vi "PH_gentec_Powermeter.panel.vi"(0 "object ref":refnum<vi>, 5 "error in (no error)":errorcluster) -> (19 "error out":errorcluster)   [LabVIEW 2014, in "PH_gentec_Powermeter.lvlib"]
doc: "By this VI apowermeter can be operated. \n\nThe panel is divided into the Tab Control which contains three pages and the most important elements.\nThe 1st page of the Tab Control contains the general information Range, Trigger Level, Scaling Factor (the user can set these values), Uncorrected Value and Serial Number (these are indicators). \nThe 2nd page contains everything relevant for the Statistics Mode of the powermeter. Here you can Start/Stop the statistic data collection, set the Number of Pulses, Percentage of Pulses and the Number of Samples. The Cluster 'Statistic Data' views the evaluated statistic data.\nThe 3rd page contains the rarely needed status-information of the powermeter. The string views data like Active Sensitivity, Offset, Resolution and so on.\n\nBelow the Tab Control you can see: \n - Current Value views the value that is currently being displayed on the device's screen. The correct unit is appended.\n - Powermeter views the Device State: blue means no info\n darkgreen means off\n lightgreen means operating\n yellow means error detected\n - EXIT closes the front panel (GUI), while\n - Delete Instance disconnects and removes the instance from the PCS.\n\n\nLicense Agreement for this software:\n\nCopyright (C)\nGesellschaft für Schwerionenforschung, GSI\nPlanckstr. 1\n64291 Darmstadt\nGermany\n\nContact: D.Beck@gsi.de \n\nThis program is free software; you can redistribute it and/or modify it under the terms of the GNU General Public License as published by the Free Software Foundation; either version 2 of the license, or (at your option) any later version.\n\nThis program is distributed in the hope that it will be useful, but WITHOUT ANYW ARRANTY; without even the implied warranty of MERCHANTABILITY or FITNESS FOR A PARTICULAR PURPOSE. See the GNU General License for more details (http://www.gnu.org).\n\nGesellschaft für Schwerionenforschung, GSI\nPlanckstr. 1, 64291 Darmstadt, Germany\nFor all questions and ideas contact: M.Richter@gsi.de, H.Brand@gsi.de or D.Beck@gsi.de.\nLast update: 18-DEC-2002"
uses:
  PH_gentec_Powermeter.lvlib
  PH_StatusHandler/PH_StatusHandler.GUI element.ctl
  PH_Powermeter_BaseClass/PH_Powermeter_BaseClass.Energy.ctl
  PH_Powermeter_BaseClass/PH_Powermeter_BaseClass.Head Attributes.ctl
  PH_Powermeter_BaseClass/PH_Powermeter_BaseClass.Connection.ctl
  PH_Powermeter_BaseClass/PH_Powermeter_BaseClass.State.ctl
  non_GPL/instr.lib/gentec-SOLO-PE/Driver/Type Defs/gentec-SOLO-PE.Configuration Values.ctl
  non_GPL/instr.lib/gentec-SOLO-PE/Driver/Type Defs/gentec-SOLO-PE.Scale.ctl
  non_GPL/instr.lib/gentec-SOLO-PE/Driver/Type Defs/gentec-SOLO-PE.Statistics Data.ctl
  non_GPL/instr.lib/gentec-SOLO-PE/Driver/Type Defs/gentec-SOLO-PE.Data Sampling Settings.ctl
  PH_gentec_Powermeter.Sets.ctl
  PH_Powermeter_BaseClass/PH_gentec_BaseClass.Head Settings.ctl
  PH_Powermeter_BaseClass/PH_Powermeter_BaseClass.GUI Refs.ctl
  CSCore/CSObj/CSObj.lvlib
  CSCore/CSSystem/CSSystemLib/CSSystemLib.lvlib
  PH_Common/PH_Common.lvlib
  PH_Class/PH_Class.lvlib
  PH_Powermeter_BaseClass/PH_Powermeter_BaseClass.lvlib
  PH_StatusHandler/PH_StatusHandler.lvlib
  non_GPL/instr.lib/gentec-SOLO-PE/gentec-SOLO-PE - Driver.lvlib
panel:
  out "Status":T1
  out "PSDB Status":u32(colorbox)=6618880 caption="PSDB"
  in  "Tab Control":T2(tab)
  in  "Scaling Factor":dbl=1.0
  in  "Range":u32(ring) items=["Scale 1", "Scale 2", "Scale 3"]
  in  "Wavelength":u32=1 caption="nm"
  in  "Trigger Level":dbl caption="%"
  in  "Set Zero":bool
  out "Energy evolution":dbl(graph)
  out "Energy":T3={"current Value"=0.0, "unscaled"=0.0, "Scaling Factor"=1.0} {"unscaled" format="%#_6p"; "current Value" format="%#.1p"}
  in  "Start/Stop Statistics":bool caption="Start/Stop"
  in  "Data Sampling Settings":T4 {"Time Stamp" items=["Off", "On"]; "Total Duration Unit" items=["Period", "Seconds", "Minutes", "Hours", "Days", "Weeks", "Continuous", "# of Points"]; "Total Duration" max=300 step=1; "Sample Period Unit" items=["Seconds", "Minutes", "Hours", "Days", "Weeks", "Pulses"]; "Sample Rate Unit" items=["per Second", "per Minute", "per Hour", "per Day", "% pulses"]; "Sample Rate" max=300 step=1}
  out "Statistic Data":T5 {"Uncorrected Value" format="%.6f"; "Rep Rate" format="%.2f"; "Average Power" format="%.6f"; "PTP Stability" format="%.6f"; "RMS Stability" format="%.6f"; "Standard Deviation" format="%.6f"; "Average" format="%.6f"; "Minimum" format="%.6f"; "Maximum" format="%.6f"; "Current Value" format="%.6f"}
  out "Configuration Values":T6 {"Reference Value" format="%.6f"; "Lower Bond" format="%.6f"; "Upper Bound" format="%.6f"; "Resolution" format="%.7f"; "Max energy (Joulemeter)" format="%.6f"; "Max Power (Joulemeter)" format="%.6f"; "Offset 2" format="%.6f"; "Multiplier 2" format="%.6f"; "Offset 1" format="%.6f"; "Multiplier 1" format="%.6f"; "Zero Offset" format="%.6f"; "Trig Level" format="%.6f"; "Current Scale" items=["Auto", "1 pJ", "3 pJ", "10 pJ", "30 pJ", "100 pJ", "300 pJ", "1 nJ", "3 nJ", "10 nJ", "30 nJ", "100 nJ", "300 nJ", "1 uJ", "3 uJ", "10 uJ", "30 uJ", "100 uJ", "300 uJ", "1 mJ", "3 mJ", "10 mJ", "30 mJ", "100 mJ", "300 mJ", "1 J", "3 J", "10 J", "30 J", "100 J", "300 J", "1 kJ", "3 kJ", "10 kJ", "30 kJ", "100 kJ", "300 kJ", "1 MJ", "3 MJ", "10 MJ", "30 MJ", "100 MJ", "300 MJ"]; "Scale Max Energy" items=["Auto", "1 pJ", "3 pJ", "10 pJ", "30 pJ", "100 pJ", "300 pJ", "1 nJ", "3 nJ", "10 nJ", "30 nJ", "100 nJ", "300 nJ", "1 uJ", "3 uJ", "10 uJ", "30 uJ", "100 uJ", "300 uJ", "1 mJ", "3 mJ", "10 mJ", "30 mJ", "100 mJ", "300 mJ", "1 J", "3 J", "10 J", "30 J", "100 J", "300 J", "1 kJ", "3 kJ", "10 kJ", "30 kJ", "100 kJ", "300 kJ", "1 MJ", "3 MJ", "10 MJ", "30 MJ", "100 MJ", "300 MJ"]; "Scale Min Energy" items=["Auto", "1 pJ", "3 pJ", "10 pJ", "30 pJ", "100 pJ", "300 pJ", "1 nJ", "3 nJ", "10 nJ", "30 nJ", "100 nJ", "300 nJ", "1 uJ", "3 uJ", "10 uJ", "30 uJ", "100 uJ", "300 uJ", "1 mJ", "3 mJ", "10 mJ", "30 mJ", "100 mJ", "300 mJ", "1 J", "3 J", "10 J", "30 J", "100 J", "300 J", "1 kJ", "3 kJ", "10 kJ", "30 kJ", "100 kJ", "300 kJ", "1 MJ", "3 MJ", "10 MJ", "30 MJ", "100 MJ", "300 MJ"]; "Active Sensitivity" format="%.6f"; "Calibration Sensitivity" format="%.6f"}
  out "Current Settings":T8={"Trigger Level"=0.0, "Wavelength"=1, "Range"=0}
  out "Wanted Settings":T8={"Trigger Level"=0.0, "Wavelength"=1, "Range"=0}
  out "Wanted Sets":T9 {"Data Sampling Settings"."Time Stamp" items=["Off", "On"]; "Data Sampling Settings"."Total Duration Unit" items=["Period", "Seconds", "Minutes", "Hours", "Days", "Weeks", "Continuous", "# of Points"]; "Data Sampling Settings"."Total Duration" max=300 step=1; "Data Sampling Settings"."Sample Period Unit" items=["Seconds", "Minutes", "Hours", "Days", "Weeks", "Pulses"]; "Data Sampling Settings"."Sample Rate Unit" items=["per Second", "per Minute", "per Hour", "per Day", "% pulses"]; "Data Sampling Settings"."Sample Rate" max=300 step=1}
  out "Current Sets":T9 {"Data Sampling Settings"."Time Stamp" items=["Off", "On"]; "Data Sampling Settings"."Total Duration Unit" items=["Period", "Seconds", "Minutes", "Hours", "Days", "Weeks", "Continuous", "# of Points"]; "Data Sampling Settings"."Total Duration" max=300 step=1; "Data Sampling Settings"."Sample Period Unit" items=["Seconds", "Minutes", "Hours", "Days", "Weeks", "Pulses"]; "Data Sampling Settings"."Sample Rate Unit" items=["per Second", "per Minute", "per Hour", "per Day", "% pulses"]; "Data Sampling Settings"."Sample Rate" max=300 step=1}
  out "VISA resource":refnum<visa-resource-name>
  out "Connection":T10
  out "Head Attributes":T12={"Instrument Type"="---", "Head Version"="---", "Head Name"="---", "Serial Number"="---", "Firmware"="---", "Sensor Type"="---", "MinimumRange"=0, "Maximum Range"=0, "Min Wavelength"=-1, "Max Wavelength"=-1}
  in  "Delete":bool
  in  "Exit":bool
  # "PCS"
  # "3.40"
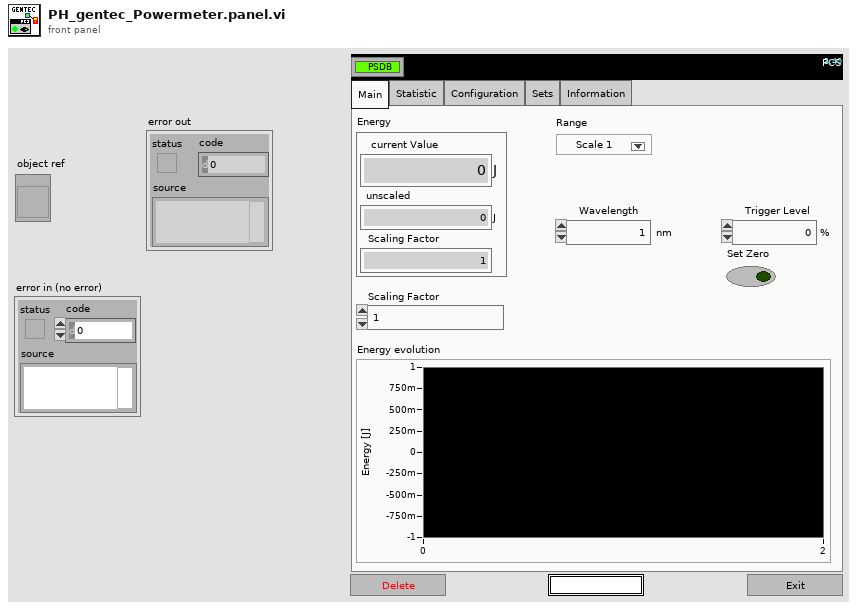
[diagram p1: front panel]
types:
  T1 = typedef "PH_StatusHandler.lvlib/PH_StatusHandler.GUI element.ctl" = u16
  T2 = enum32{"Main", "Statistic", "Configuration", "Sets", "Information"}
  T3 = typedef "PH_Powermeter_BaseClass.lvlib/PH_Powermeter_BaseClass.Energy.ctl" = cluster{"current Value":dbl, "unscaled":dbl, "Scaling Factor":dbl}
  T4 = typedef "gentec-SOLO-PE - Driver.lvlib/gentec-SOLO-PE.Data Sampling Settings.ctl" = cluster{"Sample Rate":u32, "Sample Rate Unit":u32, "Sample Period":u32, "Sample Period Unit":u32, "Total Duration":u32, "Total Duration Unit":u32, "Time Stamp":u32}
  T5 = typedef "gentec-SOLO-PE - Driver.lvlib/gentec-SOLO-PE.Statistics Data.ctl" = cluster{"Current Value":dbl, "Maximum":dbl, "Minimum":dbl, "Average":dbl, "Standard Deviation":dbl, "RMS Stability":dbl, "PTP Stability":dbl, "Current Time In Period":u32, "Total Time in Period":u32, "Pulse Number":u32, "Total Pulses":u32, "Average Power":dbl, "Rep Rate":dbl, "Uncorrected Value":dbl}
  T6 = typedef "gentec-SOLO-PE - Driver.lvlib/gentec-SOLO-PE.Configuration Values.ctl" = cluster{"Head Type":string, "Head Version":u32, "Serial Number":string, "Calibration Sensitivity":dbl, "Default Wavelength":u32, "Active Sensitivity":dbl, "Active Wavelength":u32, "Scale Min Power":u32, "Scale Max Power":u32, "Scale Min Energy":T7, "Scale Max Energy":T7, "Current Scale":T7, "Calo Mode":bool, "Anticipation":bool, "External Trig":bool, "Trig Level":dbl, "Zero Offset":dbl, "Multiplier 1":dbl, "Offset 1":dbl, "Multiplier 2":dbl, "Offset 2":dbl, "Max Power (Joulemeter)":dbl, "Max energy (Joulemeter)":dbl, "Currently Logging":bool, "Analog Out Active":bool, "Resolution":dbl, "Currently Calculating Stats":bool, "High-Resolution Display":bool, "Scale Min Wavelenght":u32, "Scale Max Wavelenght":u32, "Upper Bound":dbl, "Lower Bond":dbl, "Reference Value":dbl, "Thresholds Active":bool, "Fail":bool}
  T7 = typedef "gentec-SOLO-PE - Driver.lvlib/gentec-SOLO-PE.Scale.ctl" = u32
  T8 = typedef "PH_Powermeter_BaseClass.lvlib/PH_gentec_BaseClass.Head Settings.ctl" = cluster{"Trigger Level":dbl, "Wavelength":u32, "Range":u32}
  T9 = typedef "PH_gentec_Powermeter.lvlib/PH_gentec_Powermeter.Sets.ctl" = cluster{"Data Sampling Settings":T4, "Set Zero":bool}
  T10 = typedef "PH_Powermeter_BaseClass.lvlib/PH_Powermeter_BaseClass.Connection.ctl" = cluster{"failed checks":i8, "Timeout":bool, "Data read":string, "Failure":bool, "Error":bool, "State":T11}
  T11 = typedef "PH_Powermeter_BaseClass.lvlib/PH_Powermeter_BaseClass.State.ctl" = enum32{"off", "operating", "opened", "checked", "connected", "Sets to change", "running"}
  T12 = typedef "PH_Powermeter_BaseClass.lvlib/PH_Powermeter_BaseClass.Head Attributes.ctl" = cluster{"Instrument Type":string, "Head Version":string, "Head Name":string, "Serial Number":string, "Firmware":string, "Sensor Type":string, "MinimumRange":u32, "Maximum Range":u32, "Min Wavelength":i32, "Max Wavelength":i32}
  T13 = typedef "PH_Powermeter_BaseClass.lvlib/PH_Powermeter_BaseClass.GUI Refs.ctl" = cluster{"Head Attributes":refnum<vi>, "Energy":refnum<vi>, "Connection":refnum<vi>, "VISA Resource":refnum<vi>, "Energy evolution":refnum<vi>, "Scaling Factor":refnum<vi>, "Range":refnum<vi>, "Wavelength":refnum<vi>, "Trigger Level":refnum<vi>, "Wanted Settings":refnum<vi>, "Current Settings":refnum<vi>}
  T14 = typedef "PH_gentec_Powermeter.lvlib/PH_gentec_Powermeter.i attribute.ctl" = cluster{"GUI References":cluster{"delete":refnum<vi>, "start stop Statistics":refnum<vi>, "Statistic Data":refnum<vi>, "Configuration Values":refnum<vi>, "Set Zero":refnum<vi>, "Data Sampling Settings":refnum<vi>, "Wanted Sets":refnum<vi>, "Current Sets":refnum<vi>}, "Start Stop Statistics":bool, "Wanted Sets":T9, "Current Sets":T9}
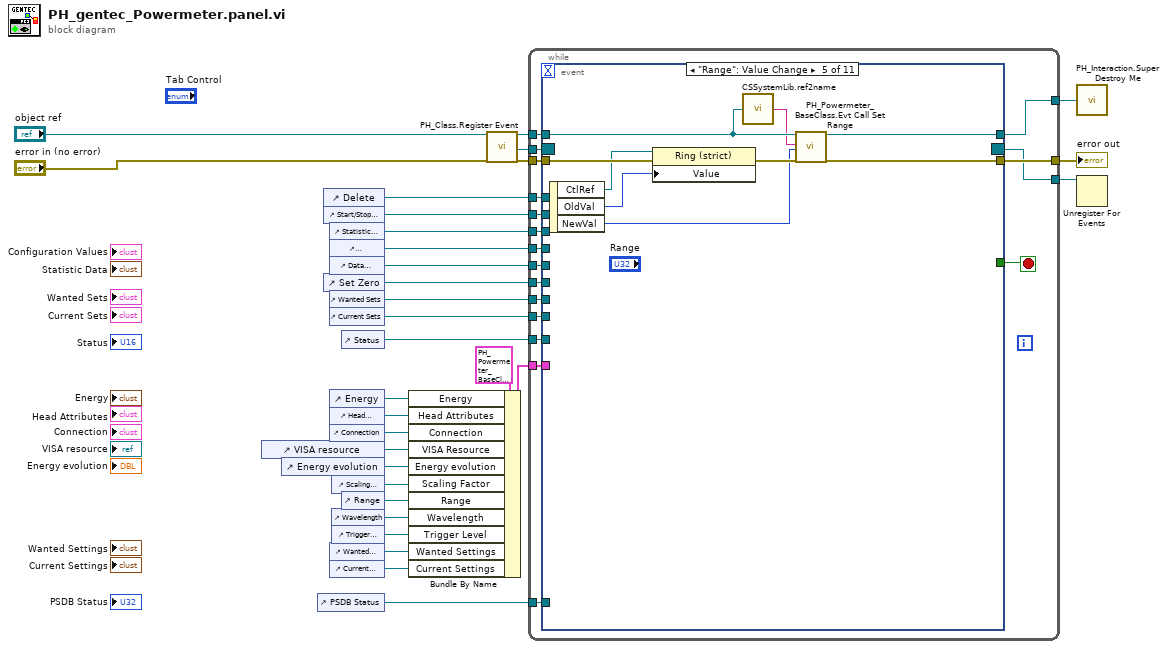
[diagram p0: block diagram]
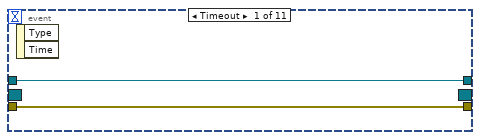
[diagram p2: hidden frame]
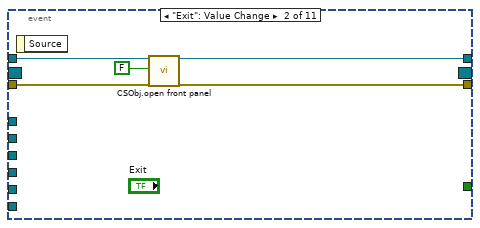
[diagram p3: hidden frame]
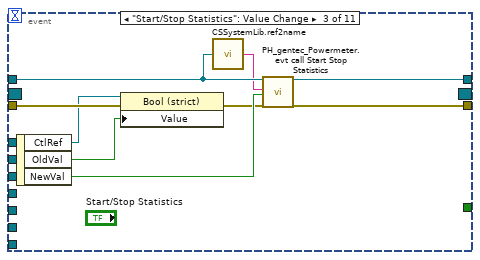
[diagram p4: hidden frame]
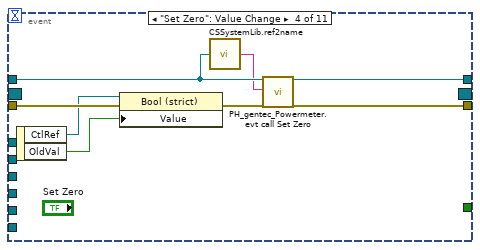
[diagram p5: hidden frame]
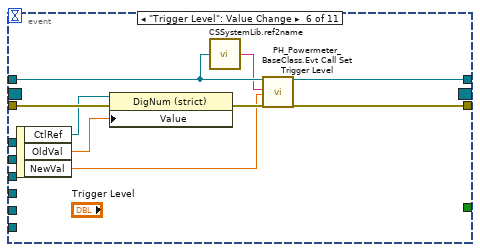
[diagram p6: hidden frame]
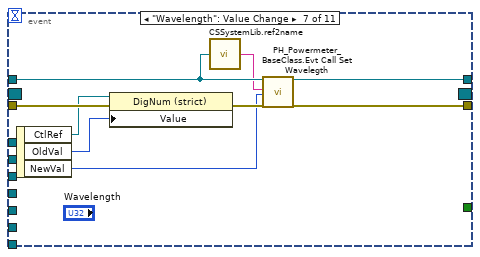
[diagram p7: hidden frame]
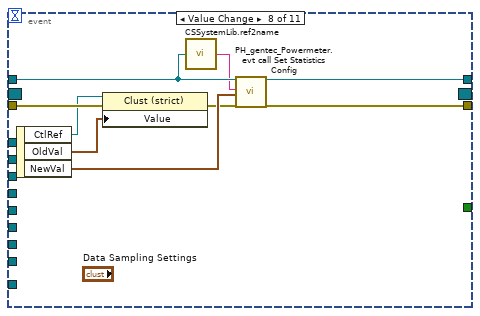
[diagram p8: hidden frame]
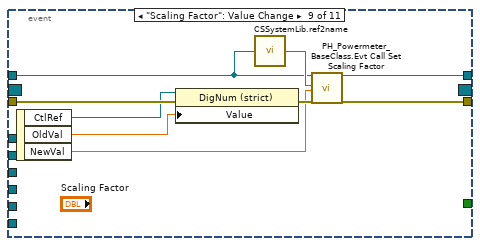
[diagram p9: hidden frame]
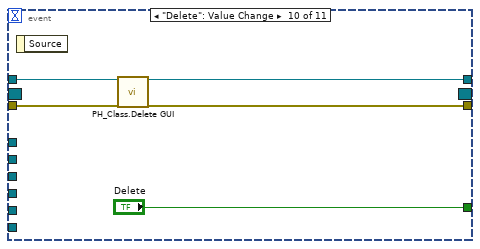
[diagram p10: hidden frame]
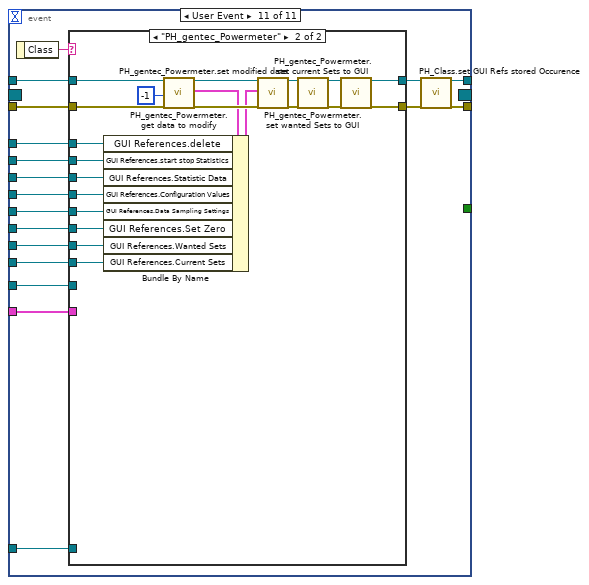
[diagram p11: hidden frame]
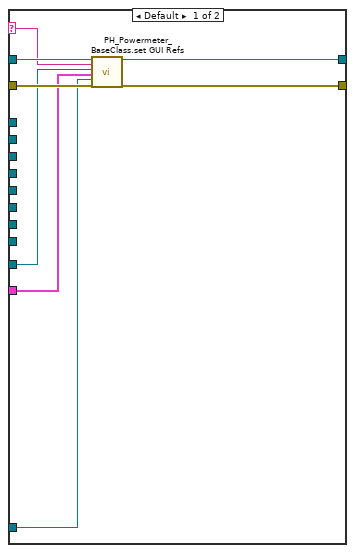
[diagram p12: hidden frame]
diagram:
  n1 = control-ref of="VISA resource"() -> (w14:refnum<vi>)
  n2 = control-ref of="Energy evolution"() -> (w9:refnum<vi>)
  n3 = control-ref of="PSDB Status"() -> (w21:refnum<vi>)
  n4 = control-ref of="Delete"() -> (w23:refnum<vi>)
  n5 = control-ref of="Start/Stop Statistics"() -> (w22:refnum<vi>)
  n6 = control-ref of="Set Zero"() -> (w13:refnum<vi>)
  n7 = control-ref of="Statistic Data"() -> (w12:refnum<vi>)
  n8 = control-ref of="Configuration Values"() -> (w11:refnum<vi>)
  n9 = control-ref of="Data Sampling Settings"() -> (w10:refnum<vi>)
  n10 = control-ref of="Wanted Sets"() -> (w2:refnum<vi>)
  n11 = control-ref of="Current Sets"() -> (w1:refnum<vi>)
  n12 = control-ref of="Energy"() -> (w17:refnum<vi>)
  n13 = control-ref of="Head Attributes"() -> (w16:refnum<vi>)
  n14 = control-ref of="Connection"() -> (w15:refnum<vi>)
  n15 = control-ref of="Wanted Settings"() -> (w7:refnum<vi>)
  n16 = control-ref of="Current Settings"() -> (w6:refnum<vi>)
  n17 = control-ref of="Scaling Factor"() -> (w8:refnum<vi>)
  n18 = control-ref of="Wavelength"() -> (w4:refnum<vi>)
  n19 = control-ref of="Trigger Level"() -> (w5:refnum<vi>)
  n20 = control-ref of="Status"() -> (w20:refnum<vi>)
  n21 = control-ref of="Range"() -> (w3:refnum<vi>)
  n22 = Bundle By Name(cluster=T13 {"Head Attributes"=refnum, "Energy"=refnum, "Connection"=refnum, "VISA Resource"=refnum, "Energy evolution"=refnum, "Scaling Factor"=refnum, "Range"=refnum, "Wavelength"=refnum, "Trigger Level"=refnum, "Wanted Settings"=refnum, "Current Settings"=refnum} ("Powermeter Base Class GUI References"), "Energy"=w17, "Head Attributes"=w16, "Connection"=w15, "VISA Resource"=w14, "Energy evolution"=w9, "Scaling Factor"=w8, "Range"=w3, "Wavelength"=w4, "Trigger Level"=w5, "Wanted Settings"=w7, "Current Settings"=w6) -> (w18:T13)
  n23 = call "PH_Class.Register Event.vi"("i ref in"="object ref", "error in (no error)"="error in (no error)") -> ("i ref out"=w29:refnum<vi>, "Event Registration Refnum"=w27:refnum<event-registration>, "error out"=w28:errorcluster)  [unwired: 15 in]
  n24 = while {
    tunnel: w29 -> [w46]
    tunnel: [w45] -> w30
    tunnel: w28 -> [w48]
    tunnel: [w47] -> w31
    tunnel: w27 -> [w44]
    tunnel: [w43] -> w26
    tunnel: w23 -> [w42]
    tunnel: w22 -> [w41]
    tunnel: w12 -> [w40]
    tunnel: w11 -> [w39]
    tunnel: w10 -> [w38]
    tunnel: w21 -> [w37]
    tunnel: w20 -> [w36]
    tunnel: w18 -> [w35]
    tunnel: w13 -> [w34]
    tunnel: w2 -> [w33]
    tunnel: w1 -> [w32]
    stop <- w49 stop-if-true
    n25 = event shown="[4] \"Range\": Value Change" {
      selector: w44 -> [_ _ _ _ _ _ _ _ _ _ _]
      dyn-events: [_ _ _ _ _ _ _ _ _ _ _] -> w43
      timeout: _ -> [_ _ _ _ _ _ _ _ _ _ _]
      tunnel: [_ _ _ _ _ _ _ _ _ "Delete" _] -> w49
      tunnel: w46 -> [w50 w56 w61 w71 w80 w89 w98 w106 w116 w121 w141]
      tunnel: w48 -> [w51 w54 w64 w69 w78 w87 w96 w109 w115 w122 w140]
      tunnel: [w51 w53 w63 w73 w82 w91 w100 w108 w114 w119 w136] -> w47
      tunnel: [w50 w52 w62 w72 w81 w90 w99 w107 w113 w120 w137] -> w45
      tunnel: w42 -> [_ _ _ _ _ _ _ _ _ _ w135]
      tunnel: w41 -> [_ _ _ _ _ _ _ _ _ _ w134]
      tunnel: w40 -> [_ _ _ _ _ _ _ _ _ _ w133]
      tunnel: w39 -> [_ _ _ _ _ _ _ _ _ _ w132]
      tunnel: w38 -> [_ _ _ _ _ _ _ _ _ _ w131]
      tunnel: w37 -> [_ _ _ _ _ _ _ _ _ _ w129]
      tunnel: w36 -> [_ _ _ _ _ _ _ _ _ _ w128]
      tunnel: w35 -> [_ _ _ _ _ _ _ _ _ _ w127]
      tunnel: w34 -> [_ _ _ _ _ _ _ _ _ _ w126]
      tunnel: w33 -> [_ _ _ _ _ _ _ _ _ _ w125]
      tunnel: w32 -> [_ _ _ _ _ _ _ _ _ _ w124]
      event Timeout {
        n26 = event-data() -> ()  [unwired: 1 in, 2 out]
      }
      event "Exit": Value Change {
        n27 = event-data() -> ()  [unwired: 1 in, 1 out]
        n28 = call "CSObj.open front panel.vi"("i ref in"=w56, "frontPanelOpen"=FALSE ("front panel open"), "error in (no error)"=w54) -> ("i ref out"=w52:refnum<vi>, "error out"=w53:errorcluster)  [unwired: 15 in]
      }
      event "Start/Stop Statistics": Value Change {
        n29 = event-data() -> ("CtlRef"=w58:refnum<vi>, "OldVal"=w57:bool, "NewVal"=w65:bool)  [unwired: 1 in]
        n30 = property class="Bool (strict)"(reference=w58, error in=w64, "Value"=w57) -> (error out=w59:errorcluster)  [unwired: 1 out]
        n31 = call "CSSystemLib.ref2name.vi"("obj refnum"=w61) -> ("name"=w60:string)
        n32 = call "PH_gentec_Powermeter.evt call Start Stop Statistics.vi"("i ref in"=w61, "Instance"=w60, "Start/Stop Statistics"=w65, "error in (no error)"=w59) -> ("i ref out"=w62:refnum<vi>, "error out"=w63:errorcluster)  [unwired: 14 in]
      }
      event "Set Zero": Value Change {
        n33 = event-data() -> ("CtlRef"=w67:refnum<vi>, "OldVal"=w66:bool)  [unwired: 1 in]
        n34 = property class="Bool (strict)"(reference=w67, error in=w69, "Value"=w66) -> (error out=w68:errorcluster)  [unwired: 1 out]
        n35 = call "CSSystemLib.ref2name.vi"("obj refnum"=w71) -> ("name"=w70:string)
        n36 = call "PH_gentec_Powermeter.evt call Set Zero.vi"("i ref in"=w71, "Instance"=w70, "error in (no error)"=w68) -> ("i ref out"=w72:refnum<vi>, "error out"=w73:errorcluster)  [unwired: 15 in]
      }
      event "Range": Value Change {
        n37 = event-data() -> ("CtlRef"=w77:refnum<vi>, "OldVal"=w76:u32, "NewVal"=w74:u32)  [unwired: 1 in]
        n38 = property class="Ring (strict)"(reference=w77, error in=w78, "Value"=w76) -> (error out=w75:errorcluster)  [unwired: 1 out]
        n39 = call "CSSystemLib.ref2name.vi"("obj refnum"=w80) -> ("name"=w79:string)
        n40 = call "PH_Powermeter_BaseClass.Evt Call Set Range.vi"("i ref in"=w80, "Instance"=w79, "Range"=w74, "error in (no error)"=w75) -> ("i ref out"=w81:refnum<vi>, "error out"=w82:errorcluster)  [unwired: 14 in]
      }
      event "Trigger Level": Value Change {
        n41 = event-data() -> ("CtlRef"=w86:refnum<vi>, "OldVal"=w85:dbl, "NewVal"=w83:dbl)  [unwired: 1 in]
        n42 = property class="DigNum (strict)"(reference=w86, error in=w87, "Value"=w85) -> (error out=w84:errorcluster)  [unwired: 1 out]
        n43 = call "CSSystemLib.ref2name.vi"("obj refnum"=w89) -> ("name"=w88:string)
        n44 = call "PH_Powermeter_BaseClass.Evt Call Set Trigger Level.vi"("i ref in"=w89, "Instance"=w88, "Scaling Factor"=w83, "error in (no error)"=w84) -> ("i ref out"=w90:refnum<vi>, "error out"=w91:errorcluster)  [unwired: 14 in]
      }
      event "Wavelength": Value Change {
        n45 = event-data() -> ("CtlRef"=w95:refnum<vi>, "OldVal"=w94:u32, "NewVal"=w92:u32)  [unwired: 1 in]
        n46 = property class="DigNum (strict)"(reference=w95, error in=w96, "Value"=w94) -> (error out=w93:errorcluster)  [unwired: 1 out]
        n47 = call "CSSystemLib.ref2name.vi"("obj refnum"=w98) -> ("name"=w97:string)
        n48 = call "PH_Powermeter_BaseClass.Evt Call Set Wavelegth.vi"("i ref in"=w98, "Instance"=w97, "Scaling Factor"=w92, "error in (no error)"=w93) -> ("i ref out"=w99:refnum<vi>, "error out"=w100:errorcluster)  [unwired: 14 in]
      }
      event Value Change {
        n49 = event-data() -> ("CtlRef"=w102:refnum<vi>, "OldVal"=w101:T4, "NewVal"=w104:T4)  [unwired: 1 in]
        n50 = property class="Clust (strict)"(reference=w102, error in=w109, "Value"=w101) -> (error out=w103:errorcluster)  [unwired: 1 out]
        n51 = call "CSSystemLib.ref2name.vi"("obj refnum"=w106) -> ("name"=w105:string)
        n52 = call "PH_gentec_Powermeter.evt call Set Statistics Config.vi"("i ref in"=w106, "Instance"=w105, "Number Of Pulses"=w104, "error in (no error)"=w103) -> ("i ref out"=w107:refnum<vi>, "error out"=w108:errorcluster)  [unwired: 14 in]
      }
      event "Scaling Factor": Value Change {
        n53 = event-data() -> ("CtlRef"=w112:refnum<vi>, "OldVal"=w111:dbl, "NewVal"=w110:dbl)  [unwired: 1 in]
        n54 = property class="DigNum (strict)"(reference=w112, error in=w115, "Value"=w111) -> (error out=w117:errorcluster)  [unwired: 1 out]
        n55 = call "CSSystemLib.ref2name.vi"("obj refnum"=w116) -> ("name"=w118:string)
        n56 = call "PH_Powermeter_BaseClass.Evt Call Set Scaling Factor.vi"("i ref in"=w116, "Instance"=w118, "Scaling Factor"=w110, "error in (no error)"=w117) -> ("i ref out"=w113:refnum<vi>, "error out"=w114:errorcluster)  [unwired: 14 in]
      }
      event "Delete": Value Change {
        n57 = event-data() -> ()  [unwired: 1 in, 1 out]
        n58 = call "PH_Class.Delete GUI.vi"("VI in"=w121, "error in (no error)"=w122) -> ("VI out"=w120:refnum<vi>, "error out"=w119:errorcluster)  [unwired: 16 in]
      }
      event User Event {
        n59 = event-data() -> ("Class"=w130:string)  [unwired: 1 in]
        n60 = case shown="\"PH_gentec_Powermeter\"" w130 {
          selector: w130 -> [w147 _]
          tunnel: w141 -> [w148 w166]
          tunnel: w140 -> [w149 w165]
          tunnel: [w144 w150] -> w139
          tunnel: [w145 w151] -> w138
          tunnel: w135 -> [_ w164]
          tunnel: w134 -> [_ w163]
          tunnel: w133 -> [_ w160]
          tunnel: w132 -> [_ w162]
          tunnel: w131 -> [_ w158]
          tunnel: w129 -> [w143 _]
          tunnel: w128 -> [w146 _]
          tunnel: w127 -> [w142 _]
          tunnel: w126 -> [_ w159]
          tunnel: w125 -> [_ w157]
          tunnel: w124 -> [_ w156]
          frame Default {
            n61 = call "PH_Powermeter_BaseClass.set GUI Refs.vi"("VI in"=w148, "Class"=w147, "Status GUI Reference"=w146, "Powermeter Base Class GUI References"=w142, "PSDB Status GUI Reference"=w143, "error in (no error)"=w149) -> ("VI out"=w145:refnum<vi>, "error out"=w144:errorcluster)  [unwired: 12 in]
          }
          frame "PH_gentec_Powermeter" {
            n62 = call "PH_gentec_Powermeter.get data to modify.vi"("i ref in"=w166, "ms timeout (10000)"=-1, "error in (no error)"=w165) -> ("i ref out"=w170:refnum<vi>, "i attribute"=w167:T14, "error out"=w169:errorcluster)  [unwired: 13 in, 1 out]
            n63 = Bundle By Name(cluster=w167, "GUI References.delete"=w164, "GUI References.start stop Statistics"=w163, "GUI References.Statistic Data"=w160, "GUI References.Configuration Values"=w162, "GUI References.Data Sampling Settings"=w158, "GUI References.Set Zero"=w159, "GUI References.Wanted Sets"=w157, "GUI References.Current Sets"=w156) -> (w161:T14)
            n64 = call "PH_gentec_Powermeter.set modified data.vi"("i ref in"=w170, "i attribute"=w161, "error in (no error)"=w169) -> ("i ref out"=w152:refnum<vi>, "error out"=w153:errorcluster)  [unwired: 15 in]
            n65 = call "PH_gentec_Powermeter.set wanted Sets to GUI.vi"("i ref in"=w152, "error in"=w153) -> ("i ref out"=w155:refnum<vi>, "error out"=w154:errorcluster)  [unwired: 16 in]
            n66 = call "PH_gentec_Powermeter.set current Sets to GUI.vi"("i ref in"=w155, "error in"=w154) -> ("i ref out"=w151:refnum<vi>, "error out"=w150:errorcluster)  [unwired: 16 in]
          }
        }
        n67 = call "PH_Class.set GUI Refs stored Occurence.vi"("i ref in"=w138, "error in (no error)"=w139) -> ("i ref out"=w137:refnum<vi>, "error out"=w136:errorcluster)  [unwired: 16 in]
      }
    }
  }
  "error out" <- w31
  n68 = call "PH_Interaction.Super Destroy Me.vi"("i ref out"=w30) -> ()
  n69 = Unregister For Events(event registration refnum=w26) -> ()  [unwired: 1 in, 1 out]
